vi "makeTcpCommand64bit.vi"(8 "error in":errorcluster, 10 "Variant":variant, 11 "Command":T1) -> (0 "error out":errorcluster, 2 "size":i32, 3 "String":string)   [LabVIEW 2018]
uses:
  control/enumTcpCommand.ctl
  control/enumFgvFunction.ctl
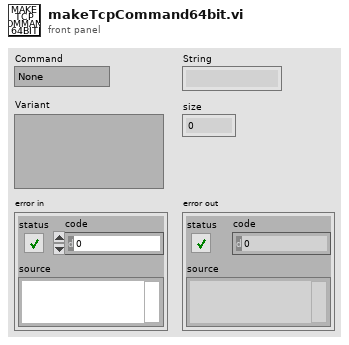
[diagram p1: front panel]
types:
  T1 = typedef "enumTcpCommand.ctl" = enum16{"None", "Stop", "E-Stop", "Set Position Control Mode", "Set Jog Control Mode", "Set Control Mode", "Set Jog Control Profile Parameter", "Set Position Control Profile Parameter", "Set Jog State", "Set Position", "Start Position Control", "Get Total State", "Get Platform State", "Get Sensor State", "Get Position State", "Init Platform"}
  T2 = typedef "enumFgvFunction.ctl" = enum16{"Open", "Read", "Check", "Write", "Close"}
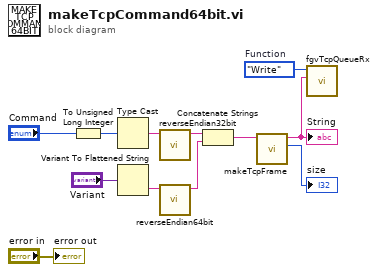
[diagram p0: block diagram]
diagram:
  w7 = enumFgvFunction."Write"  # Function
  n1 = To Unsigned Long Integer(number="Command") -> (unsigned 32bit integer=w12:u32)
  n2 = Type Cast(x=w12) -> (*(type *) &x=w5:string)  [unwired: 1 in]
  n3 = Variant To Flattened String(Variant="Variant") -> (data string=w2:string)  [unwired: 1 out]
  n4 = call "reverseEndian32bit.vi"("In"=w5) -> ("Out"=w4:string)  [unwired: 9 in, 1 out]
  n5 = call "reverseEndian64bit.vi"("In"=w2) -> ("Out"=w1:string)  [unwired: 9 in, 1 out]
  n6 = Concatenate Strings(w4, w1) -> (w3:string)
  n7 = call "makeTcpFrame.vi"("String in"=w3) -> ("size"=→"size":i32, "String out"=w6:string)  [unwired: 8 in, 1 out]
  "String" <- w6
  n8 = call "fgvTcpQueueRx.vi"("Write"=w6, "Function"=w7) -> ()  [unwired: 7 in, 3 out]
  "error out" <- "error in"
